vi "TEMOCR-Start Phase.vi"(0 "AO in":T1, 2 "SGDA Queue":refnum<queue>, 9 "ProgressBar":refnum<vi>, 11 "error in (no error)":errorcluster, 12 "seqStep":i32, 13 "phase":i32) -> (4 "AO out":T1, 14 "Step":T2, 15 "error out":errorcluster)   [LabVIEW 2015]
uses:
  Typedefs/TEMOCR-Sequence Step.ctl
  Typedefs/TEMOCR-AO Data.ctl
  Typedefs/TEMOCR-Parameters.ctl
  Typedefs/TEMOCR-Probe.ctl
  Typedefs/TEMOCR-Elicitor.ctl
  Human Studies/SFM Frontend/LV Source/Typedefs/HSTS-Transducer.ctl
  Typedefs/TEMOCR-Sequence.ctl
  Typedefs/TEMOCR-Analysis.ctl
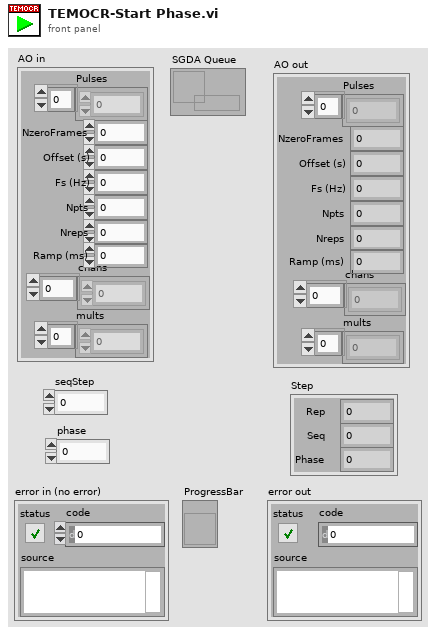
[diagram p1: front panel]
types:
  T1 = typedef "TEMOCR-AO Data.ctl" = cluster{"Pulses":dbl[], "Fs (Hz)":dbl, "Npts":i32, "mults":dbl[], "chans":i32[], "Nreps":i32, "NzeroFrames":i32, "Offset (s)":dbl, "Ramp (ms)":dbl}
  T2 = typedef "TEMOCR-Sequence Step.ctl" = cluster{"Rep":i32, "Seq":i32, "Phase":i32}
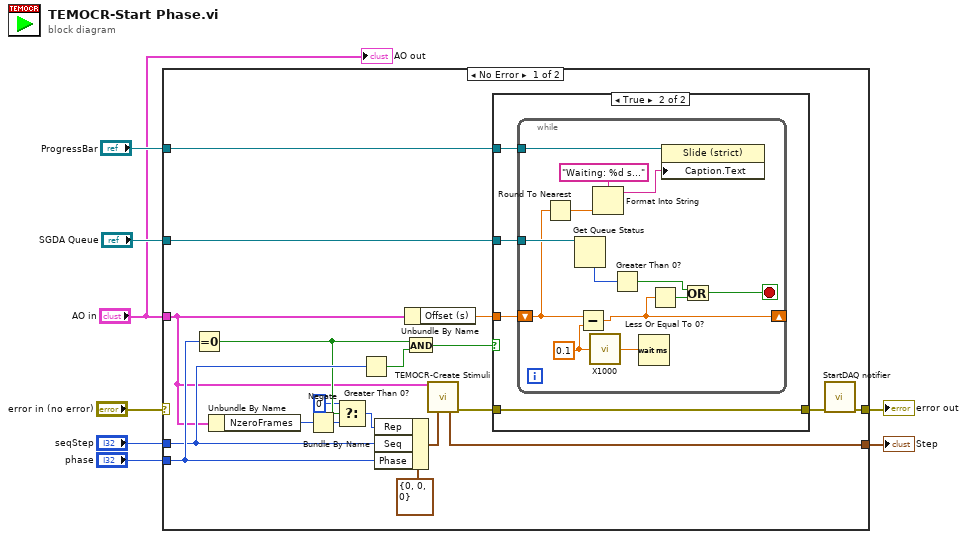
[diagram p0: block diagram]
diagram:
  n1 = case shown="No Error" "error in (no error)" {
    selector: "error in (no error)" -> [_ w46]
    tunnel: [w25 _] -> w8
    tunnel: "phase" -> [w24 _]
    tunnel: "seqStep" -> [w23 _]
    tunnel: "SGDA Queue" -> [w19 _]
    tunnel: "ProgressBar" -> [w18 _]
    tunnel: [w15 w46] -> w3
    tunnel: "AO in" -> [w12 _]
    frame No Error {
      n2 = Equal To 0?(x=w24) -> (x = 0?=w14:bool)
      n3 = Unbundle By Name(w12) -> ("NzeroFrames"=w10:i32)
      n4 = Negate(x=w10) -> (-x=w9:i32)
      n5 = Select(t=0 ("f"), s=w14, f=w9) -> (s? t:f=w13:i32)
      n6 = Greater Than 0?(x=w23) -> (x > 0?=w22:bool)
      n7 = Bundle By Name(cluster=T2 {"Rep"=0, "Seq"=0, "Phase"=0} ("Step"), "Rep"=w13, "Seq"=w23, "Phase"=w24) -> (w26:T2)
      n8 = Unbundle By Name(w12) -> ("Offset (s)"=w20:dbl)
      n9 = And(x=w14, y=w22) -> (x .and. y?=w21:bool)
      n10 = call "TEMOCR-Create Stimuli.vi"("AO"=w12, "Step In"=w26) -> ("Step"=w25:T2, "error out"=w17:errorcluster)  [unwired: 11 in, 1 out]
      n11 = case shown="True" w21 {
        tunnel: w20 -> [_ w31]
        tunnel: w19 -> [_ w32]
        tunnel: w18 -> [_ w30]
        tunnel: w17 -> [w28 w29]
        tunnel: [w28 w29] -> w16
        frame False {
        }
        frame True {
          n12 = while {
            tunnel: w32 -> [w45]
            shift-right: [w44] -> _
            shift-left: w31 -> [w37]
            tunnel: w30 -> [w34]
            stop <- w40 stop-if-true
            w38 = 0.1
            n13 = Round To Nearest(number=w37) -> (nearest integer value=w36:dbl)
            n14 = Get Queue Status(queue=w45) -> (# elements in queue=w43:i32)  [unwired: 2 in, 7 out]
            n15 = Subtract(x=w37, y=w38) -> (x-y=w44:dbl)
            n16 = call "X1000.vi"("X"=w38) -> ("X/1000"=w39:dbl)
            n17 = Format Into String(format string="Waiting: %d s...", w36) -> (resulting string=w33:string)  [unwired: 2 in, 1 out]
            n18 = Greater Than 0?(x=w43) -> (x > 0?=w41:bool)
            n19 = Wait (ms)(milliseconds to wait=w39) -> ()  [unwired: 1 out]
            n20 = Less Or Equal To 0?(x=w44) -> (x <= 0?=w42:bool)
            n21 = property class="Slide (strict)"(reference=w34, "Caption.Text"=w33) -> ()  [unwired: 1 in, 2 out]
            n22 = Or(x=w41, y=w42) -> (x .or. y?=w40:bool)
          }
        }
      }
      n23 = call "StartDAQ notifier.vi"("error in (no error)"=w16) -> ("error out"=w15:errorcluster)  [unwired: 6 in]
    }
    frame Error {
    }
  }
  "Step" <- w8
  "error out" <- w3
  "AO out" <- "AO in"
